vi "nanocal -- nuclear schottky fit V7.vi"() -> ()   [LabVIEW 2021] (continued)
0494_220602_RAW_cal__ref_\" ->   <|    \"ζ\" -> 0.158252879790   ,  \"τ1\" -> 0.024827950008   ,  \"τS\" -> 0.060146890842   ,  \"τN\" -> 0.015050943013   ,  \"τC\" -> 0.000951750255   ,  \"κ0\" -> 0.000000001243   ,  \"mm1\" -> 0.000128517617   ,  \"mm2\" -> 0.018585917114   ,  \"mm3\" -> 0.094163373149   ,  \"T\" -> 0.250000000000   ,  \"B\" -> 8.000000000000   ,  \"θ\" -> 45.000000000000   ,  \"Reoff\" -> -20024489.795918367800   ,  \"Imoff\" -> 0.000000000000   ,  \"στ1\" -> 0.008614865267   ,  \"στS\" -> 0.002364789587   ,  \"στN\" -> 0.002490160339    |>   , \n\"IDS0494_220602_RAW_cal__sam_\" ->   <|    \"ζ\" -> 0.000000000000   ,  \"τ1\" -> 0.000000000000   ,  \"τS\" -> 0.000000000000   ,  \"τN\" -> 0.000000000000   ,  \"τC\" -> 0.000000000000   ,  \"κ0\" -> 0.000000000000   ,  \"mm1\" -> 0.000000000000   ,  \"mm2\" -> 0.000000000000   ,  \"mm3\" -> 0.000000000000   ,  \"T\" -> 0.250000000000   ,  \"B\" -> 8.000000000000   ,  \"θ\" -> 45.000000000000   ,  \"Reoff\" -> 0.000000000000   ,  \"Imoff\" -> 0.000000000000   ,  \"στ1\" -> 0.000000000000   ,  \"στS\" -> 0.000000000000   ,  \"στN\" -> 0.000000000000    |>   , \n\"IDS0495_220602_RAW_cal__ref_\" ->   <|    \"ζ\" -> 0.620326639374   ,  \"τ1\" -> 0.043464597459   ,  \"τS\" -> 0.134106398601   ,  \"τN\" -> 0.331630286291   ,  \"τC\" -> 0.000791545838   ,  \"κ0\" -> 0.000000000449   ,  \"mm1\" -> 0.000302343125   ,  \"mm2\" -> 0.012035033998   ,  \"mm3\" -> 0.786564323638   ,  \"T\" -> 0.120000000000   ,  \"B\" -> 8.000000000000   ,  \"θ\" -> 45.000000000000   ,  \"Reoff\" -> -197355102.040816367000   ,  \"Imoff\" -> 0.000000000000   ,  \"στ1\" -> 0.040479747535   ,  \"στS\" -> 0.067583774677   ,  \"στN\" -> 0.126300079114    |>   , \n\"IDS0495_220602_RAW_cal__sam_\" ->   <|    \"ζ\" -> 0.000000000000   ,  \"τ1\" -> 0.000000000000   ,  \"τS\" -> 0.000000000000   ,  \"τN\" -> 0.000000000000   ,  \"τC\" -> 0.000000000000   ,  \"κ0\" -> 0.000000000000   ,  \"mm1\" -> 0.000000000000   ,  \"mm2\" -> 0.000000000000   ,  \"mm3\" -> 0.000000000000   ,  \"T\" -> 0.120000000000   ,  \"B\" -> 8.000000000000   ,  \"θ\" -> 45.000000000000   ,  \"Reoff\" -> 0.000000000000   ,  \"Imoff\" -> 0.000000000000   ,  \"στ1\" -> 0.000000000000   ,  \"στS\" -> 0.000000000000   ,  \"στN\" -> 0.000000000000    |>   , \n\"IDS0496_220602_RAW_cal__ref_\" ->   <|    \"ζ\" -> 0.427468854343   ,  \"τ1\" -> 0.039705721457   ,  \"τS\" -> 0.111520336177   ,  \"τN\" -> 0.118737423491   ,  \"τC\" -> 0.000757643682   ,  \"κ0\" -> 0.000000000613   ,  \"mm1\" -> 0.000226123834   ,  \"mm2\" -> 0.018076446652   ,  \"mm3\" -> 0.350846575050   ,  \"T\" -> 0.150000000000   ,  \"B\" -> 8.000000000000   ,  \"θ\" -> 45.000000000000   ,  \"Reoff\" -> -103289795.918367386000   ,  \"Imoff\" -> 0.000000000000   ,  \"στ1\" -> 0.024554050195   ,  \"στS\" -> 0.027075430846   ,  \"στN\" -> 0.033199054106    |>   , \n\"IDS0496_220602_RAW_cal__sam_\" ->   <|    \"ζ\" -> 0.000000000000   ,  \"τ1\" -> 0.000000000000   ,  \"τS\" -> 0.000000000000   ,  \"τN\" -> 0.000000000000   ,  \"τC\" -> 0.000000000000   ,  \"κ0\" -> 0.000000000000   ,  \"mm1\" -> 0.000000000000   ,  \"mm2\" -> 0.000000000000   ,  \"mm3\" -> 0.000000000000   ,  \"T\" -> 0.150000000000   ,  \"B\" -> 8.000000000000   ,  \"θ\" -> 45.000000000000   ,  \"Reoff\" -> 0.000000000000   ,  \"Imoff\" -> 0.000000000000   ,  \"στ1\" -> 0.000000000000   ,  \"στS\" -> 0.000000000000   ,  \"στN\" -> 0.000000000000    |>   , \n\"IDS0497_220603_RAW_cal__ref_\" ->   <|    \"ζ\" -> 0.332403347952   ,  \"τ1\" -> 0.033892588666   ,  \"τS\" -> 0.089882476524   ,  \"τN\" -> 0.072116867912   ,  \"τC\" -> 0.000736636997   ,  \"κ0\" -> 0.000000000736   ,  \"mm1\" -> 0.000182924179   ,  \"mm2\" -> 0.017518148856   ,  \"mm3\" -> 0.232776621520   ,  \"T\" -> 0.170000000000   ,  \"B\" -> 8.000000000000   ,  \"θ\" -> 45.000000000000   ,  \"Reoff\" -> -72616326.530612289900   ,  \"Imoff\" -> 0.000000000000   ,  \"στ1\" -> 0.010864544003   ,  \"στS\" -> 0.009543194360   ,  \"στN\" -> 0.010830263954    |>   , \n\"IDS0497_220603_RAW_cal__sam_\" ->   <|    \"ζ\" -> 0.000000000000   ,  \"τ1\" -> 0.000000000000   ,  \"τS\" -> 0.000000000000   ,  \"τN\" -> 0.000000000000   ,  \"τC\" -> 0.000000000000   ,  \"κ0\" -> 0.000000000000   ,  \"mm1\" -> 0.000000000000   ,  \"mm2\" -> 0.000000000000   ,  \"mm3\" -> 0.000000000000   ,  \"T\" -> 0.170000000000   ,  \"B\" -> 8.000000000000   ,  \"θ\" -> 45.000000000000   ,  \"Reoff\" -> 0.000000000000   ,  \"Imoff\" -> 0.000000000000   ,  \"στ1\" -> 0.000000000000   ,  \"στS\" -> 0.000000000000   ,  \"στN\" -> 0.000000000000    |>   , \n\"IDS0498_220603_RAW_cal__ref_\" ->   <|    \"ζ\" -> 0.110734162984   ,  \"τ1\" -> 0.019381596449   ,  \"τS\" -> 0.049800010244   ,  \"τN\" -> 0.007874153241   ,  \"τC\" -> 0.001094666009   ,  \"κ0\" -> 0.000000001580   ,  \"mm1\" -> 0.000107216591   ,  \"mm2\" -> 0.015930752272   ,  \"mm3\" -> 0.068498957299   ,  \"T\" -> 0.300000000000   ,  \"B\" -> 8.000000000000   ,  \"θ\" -> 45.000000000000   ,  \"Reoff\" -> -10657142.857142858200   ,  \"Imoff\" -> 0.000000000000   ,  \"στ1\" -> 0.007394501349   ,  \"στS\" -> 0.001744107422   ,  \"στN\" -> 0.001987690041    |>   , \n\"IDS0498_220603_RAW_cal__sam_\" ->   <|    \"ζ\" -> 0.000000000000   ,  \"τ1\" -> 0.000000000000   ,  \"τS\" -> 0.000000000000   ,  \"τN\" -> 0.000000000000   ,  \"τC\" -> 0.000000000000   ,  \"κ0\" -> 0.000000000000   ,  \"mm1\" -> 0.000000000000   ,  \"mm2\" -> 0.000000000000   ,  \"mm3\" -> 0.000000000000   ,  \"T\" -> 0.300000000000   ,  \"B\" -> 8.000000000000   ,  \"θ\" -> 45.000000000000   ,  \"Reoff\" -> 0.000000000000   ,  \"Imoff\" -> 0.000000000000   ,  \"στ1\" -> 0.000000000000   ,  \"στS\" -> 0.000000000000   ,  \"στN\" -> 0.000000000000    |>   , \n\"IDS0499_220603_RAW_cal__ref_\" ->   <|    \"ζ\" -> 0.075729964973   ,  \"τ1\" -> 0.017492157350   ,  \"τS\" -> 0.042916924435   ,  \"τN\" -> 0.003910009488   ,  \"τC\" -> 0.001485143735   ,  \"κ0\" -> 0.000000001996   ,  \"mm1\" -> 0.000101508308   ,  \"mm2\" -> 0.015465208626   ,  \"mm3\" -> 0.053783720140   ,  \"T\" -> 0.360000000000   ,  \"B\" -> 8.000000000000   ,  \"θ\" -> 45.000000000000   ,  \"Reoff\" -> -3787755.102040812380   ,  \"Imoff\" -> 0.000000000000   ,  \"στ1\" -> 0.001180089795   ,  \"στS\" -> 0.000447730504   ,  \"στN\" -> 0.000150733035    |>   , \n\"IDS0499_220603_RAW_cal__sam_\" ->   <|    \"ζ\" -> 0.000000000000   ,  \"τ1\" -> 0.000000000000   ,  \"τS\" -> 0.000000000000   ,  \"τN\" -> 0.000000000000   ,  \"τC\" -> 0.000000000000   ,  \"κ0\" -> 0.000000000000   ,  \"mm1\" -> 0.000000000000   ,  \"mm2\" -> 0.000000000000   ,  \"mm3\" -> 0.000000000000   ,  \"T\" -> 0.360000000000   ,  \"B\" -> 8.000000000000   ,  \"θ\" -> 45.000000000000   ,  \"Reoff\" -> 0.000000000000   ,  \"Imoff\" -> 0.000000000000   ,  \"στ1\" -> 0.000000000000   ,  \"στS\" -> 0.000000000000   ,  \"στN\" -> 0.000000000000    |>   , \n\"IDS0500_220603_RAW_cal__ref_\" ->   <|    \"ζ\" -> 0.057062025730   ,  \"τ1\" -> 0.015621328716   ,  \"τS\" -> 0.037684759429   ,  \"τN\" -> 0.002528358408   ,  \"τC\" -> 0.001814587656   ,  \"κ0\" -> 0.000000002409   ,  \"mm1\" -> 0.000093897005   ,  \"mm2\" -> 0.014229954054   ,  \"mm3\" -> 0.045619825114   ,  \"T\" -> 0.420000000000   ,  \"B\" -> 8.000000000000   ,  \"θ\" -> 45.000000000000   ,  \"Reoff\" -> -1914285.714285716420   ,  \"Imoff\" -> 0.000000000000   ,  \"στ1\" -> 0.000955516526   ,  \"στS\" -> 0.000234895501   ,  \"στN\" -> 0.000135281330    |>   , \n\"IDS0500_220603_RAW_cal__sam_\" ->   <|    \"ζ\" -> 0.000000000000   ,  \"τ1\" -> 0.000000000000   ,  \"τS\" -> 0.000000000000   ,  \"τN\" -> 0.000000000000   ,  \"τC\" -> 0.000000000000   ,  \"κ0\" -> 0.000000000000   ,  \"mm1\" -> 0.000000000000   ,  \"mm2\" -> 0.000000000000   ,  \"mm3\" -> 0.000000000000   ,  \"T\" -> 0.420000000000   ,  \"B\" -> 8.000000000000   ,  \"θ\" -> 45.000000000000   ,  \"Reoff\" -> 0.000000000000   ,  \"Imoff\" -> 0.000000000000   ,  \"στ1\" -> 0.000000000000   ,  \"στS\" -> 0.000000000000   ,  \"στN\" -> 0.000000000000    |>   , \n\"IDS0501_220603_RAW_cal__ref_\" ->   <|    \"ζ\" -> 0.041820610943   ,  \"τ1\" -> 0.014727705147   ,  \"τS\" -> 0.032103066270   ,  \"τN\" -> 0.001402697929   ,  \"τC\" -> 0.002062288671   ,  \"κ0\" -> 0.000000003070   ,  \"mm1\" -> 0.000078146988   ,  \"mm2\" -> 0.013796091461   ,  \"mm3\" -> 0.037822751096   ,  \"T\" -> 0.520000000000   ,  \"B\" -> 8.000000000000   ,  \"θ\" -> 45.000000000000   ,  \"Reoff\" -> -1155102.040816326160   ,  \"Imoff\" -> 0.000000000000   ,  \"στ1\" -> 0.000294282186   ,  \"στS\" -> 0.000104705305   ,  \"στN\" -> 0.000024302938    |>   , \n\"IDS0501_220603_RAW_cal__sam_\" ->   <|    \"ζ\" -> 0.000000000000   ,  \"τ1\" -> 0.000000000000   ,  \"τS\" -> 0.000000000000   ,  \"τN\" -> 0.000000000000   ,  \"τC\" -> 0.000000000000   ,  \"κ0\" -> 0.000000000000   ,  \"mm1\" -> 0.000000000000   ,  \"mm2\" -> 0.000000000000   ,  \"mm3\" -> 0.000000000000   ,  \"T\" -> 0.520000000000   ,  \"B\" -> 8.000000000000   ,  \"θ\" -> 45.000000000000   ,  \"Reoff\" -> 0.000000000000   ,  \"Imoff\" -> 0.000000000000   ,  \"στ1\" -> 0.000000000000   ,  \"στS\" -> 0.000000000000   ,  \"στN\" -> 0.000000000000    |>   , \n\"IDS0502_220603_RAW_cal__ref_\" ->   <|    \"ζ\" -> 0.034670986979   ,  \"τ1\" -> 0.014178027620   ,  \"τS\" -> 0.028243061757   ,  \"τN\" -> 0.000956770293   ,  \"τC\" -> 0.002118106957   ,  \"κ0\" -> 0.000000003766   ,  \"mm1\" -> 0.000066318852   ,  \"mm2\" -> 0.013432939767   ,  \"mm3\" -> 0.033009095005   ,  \"T\" -> 0.620000000000   ,  \"B\" -> 8.000000000000   ,  \"θ\" -> 45.000000000000   ,  \"Reoff\" -> -1228571.428571428170   ,  \"Imoff\" -> 0.000000000000   ,  \"στ1\" -> 0.000460475840   ,  \"στS\" -> 0.000103102463   ,  \"στN\" -> 0.000021520778    |>   , \n\"IDS0502_220603_RAW_cal__sam_\" ->   <|    \"ζ\" -> 0.000000000000   ,  \"τ1\" -> 0.000000000000   ,  \"τS\" -> 0.000000000000   ,  \"τN\" -> 0.000000000000   ,  \"τC\" -> 0.000000000000   ,  \"κ0\" -> 0.000000000000   ,  \"mm1\" -> 0.000000000000   ,  \"mm2\" -> 0.000000000000   ,  \"mm3\" -> 0.000000000000   ,  \"T\" -> 0.620000000000   ,  \"B\" -> 8.000000000000   ,  \"θ\" -> 45.000000000000   ,  \"Reoff\" -> 0.000000000000   ,  \"Imoff\" -> 0.000000000000   ,  \"στ1\" -> 0.000000000000   ,  \"στS\" -> 0.000000000000   ,  \"στN\" -> 0.000000000000    |>   , \n\"IDS0503_220603_RAW_cal__ref_\" ->   <|    \"ζ\" -> 0.027095379561   ,  \"τ1\" -> 0.013653054815   ,  \"τS\" -> 0.022995805893   ,  \"τN\" -> 0.000444319703   ,  \"τC\" -> 0.002402226581   ,  \"κ0\" -> 0.000000005139   ,  \"mm1\" -> 0.000057649030   ,  \"mm2\" -> 0.013182559678   ,  \"mm3\" -> 0.026890317385   ,  \"T\" -> 0.820000000000   ,  \"B\" -> 8.000000000000   ,  \"θ\" -> 45.000000000000   ,  \"Reoff\" -> -959183.673469387459   ,  \"Imoff\" -> 0.000000000000   ,  \"στ1\" -> 0.001867148954   ,  \"στS\" -> 0.000121343744   ,  \"στN\" -> 0.000029055500    |>   , \n\"IDS0503_220603_RAW_cal__sam_\" ->   <|    \"ζ\" -> 0.000000000000   ,  \"τ1\" -> 0.000000000000   ,  \"τS\" -> 0.000000000000   ,  \"τN\" -> 0.000000000000   ,  \"τC\" -> 0.000000000000   ,  \"κ0\" -> 0.000000000000   ,  \"mm1\" -> 0.000000000000   ,  \"mm2\" -> 0.000000000000   ,  \"mm3\" -> 0.000000000000   ,  \"T\" -> 0.820000000000   ,  \"B\" -> 8.000000000000   ,  \"θ\" -> 45.000000000000   ,  \"Reoff\" -> 0.000000000000   ,  \"Imoff\" -> 0.000000000000   ,  \"στ1\" -> 0.000000000000   ,  \"στS\" -> 0.000000000000   ,  \"στN\" -> 0.000000000000    |>   , \n\"IDS0504_220603_RAW_cal__ref_\" ->   <|    \"ζ\" -> 0.022447798358   ,  \"τ1\" -> 0.013732237823   ,  \"τS\" -> 0.018577417913   ,  \"τN\" -> 0.000173926586   ,  \"τC\" -> 0.002459582749   ,  \"κ0\" -> 0.000000007201   ,  \"mm1\" -> 0.000047916077   ,  \"mm2\" -> 0.013432779765   ,  \"mm3\" -> 0.021883395630   ,  \"T\" -> 1.120000000000   ,  \"B\" -> 8.000000000000   ,  \"θ\" -> 45.000000000000   ,  \"Reoff\" -> -714285.714285713619   ,  \"Imoff\" -> 0.000000000000   ,  \"στ1\" -> 0.000607993232   ,  \"στS\" -> 0.000105526265   ,  \"στN\" -> 0.000003332790    |>   , \n\"IDS0504_220603_RAW_cal__sam_\" ->   <|    \"ζ\" -> 0.000000000000   ,  \"τ1\" -> 0.000000000000   ,  \"τS\" -> 0.000000000000   ,  \"τN\" -> 0.000000000000   ,  \"τC\" -> 0.000000000000   ,  \"κ0\" -> 0.000000000000   ,  \"mm1\" -> 0.000000000000   ,  \"mm2\" -> 0.000000000000   ,  \"mm3\" -> 0.000000000000   ,  \"T\" -> 1.120000000000   ,  \"B\" -> 8.000000000000   ,  \"θ\" -> 45.000000000000   ,  \"Reoff\" -> 0.000000000000   ,  \"Imoff\" -> 0.000000000000   ,  \"στ1\" -> 0.000000000000   ,  \"στS\" -> 0.000000000000   ,  \"στN\" -> 0.000000000000    |>   , \n\"IDS0505_220603_RAW_cal__ref_\" ->   <|    \"ζ\" -> 0.017603951649   ,  \"τ1\" -> 0.013742471601   ,  \"τS\" -> 0.012869162108   ,  \"τN\" -> 0.000062251305   ,  \"τC\" -> 0.002783258647   ,  \"κ0\" -> 0.000000012669   ,  \"mm1\" -> 0.000039808958   ,  \"mm2\" -> 0.013395445115   ,  \"mm3\" -> 0.016249533565   ,  \"T\" -> 1.900000000000   ,  \"B\" -> 8.000000000000   ,  \"θ\" -> 45.000000000000   ,  \"Reoff\" -> -322448.979591836221   ,  \"Imoff\" -> 0.000000000000   ,  \"στ1\" -> 0.000975208988   ,  \"στS\" -> 0.000083582947   ,  \"στN\" -> 0.000002846022    |>   , \n\"IDS0505_220603_RAW_cal__sam_\" ->   <|    \"ζ\" -> 0.000000000000   ,  \"τ1\" -> 0.000000000000   ,  \"τS\" -> 0.000000000000   ,  \"τN\" -> 0.000000000000   ,  \"τC\" -> 0.000000000000   ,  \"κ0\" -> 0.000000000000   ,  \"mm1\" -> 0.000000000000   ,  \"mm2\" -> 0.000000000000   ,  \"mm3\" -> 0.000000000000   ,  \"T\" -> 1.900000000000   ,  \"B\" -> 8.000000000000   ,  \"θ\" -> 45.000000000000   ,  \"Reoff\" -> 0.000000000000   ,  \"Imoff\" -> 0.000000000000   ,  \"στ1\" -> 0.000000000000   ,  \"στS\" -> 0.000000000000   ,  \"στN\" -> 0.000000000000    |>   , \n\"IDS0506_220603_RAW_cal__ref_\" ->   <|    \"ζ\" -> 0.017513535650   ,  \"τ1\" -> 0.013742433942   ,  \"τS\" -> 0.009294247030   ,  \"τN\" -> 0.000023643269   ,  \"τC\" -> 0.002563999230   ,  \"κ0\" -> 0.000000022469   ,  \"mm1\" -> 0.000034819598   ,  \"mm2\" -> 0.011836880672   ,  \"mm3\" -> 0.013915812404   ,  \"T\" -> 3.100000000000   ,  \"B\" -> 8.000000000000   ,  \"θ\" -> 45.000000000000   ,  \"Reoff\" -> -175510.204081632197   ,  \"Imoff\" -> 0.000000000000   ,  \"στ1\" -> 0.000768522779   ,  \"στS\" -> 0.000063413326   ,  \"στN\" -> 0.000000634158    |>   , \n\"IDS0506_220603_RAW_cal__sam_\" ->   <|    \"ζ\" -> 0.000000000000   ,  \"τ1\" -> 0.000000000000   ,  \"τS\" -> 0.000000000000   ,  \"τN\" -> 0.000000000000   ,  \"τC\" -> 0.000000000000   ,  \"κ0\" -> 0.000000000000   ,  \"mm1\" -> 0.000000000000   ,  \"mm2\" -> 0.000000000000   ,  \"mm3\" -> 0.000000000000   ,  \"T\" -> 3.100000000000   ,  \"B\" -> 8.000000000000   ,  \"θ\" -> 45.000000000000   ,  \"Reoff\" -> 0.000000000000   ,  \"Imoff\" -> 0.000000000000   ,  \"στ1\" -> 0.000000000000   ,  \"στS\" -> 0.000000000000   ,  \"στN\" -> 0.000000000000    |>   , \n\"IDS0508_220603_RAW_cal__ref_\" ->   <|    \"ζ\" -> 0.243281471751   ,  \"τ1\" -> 0.025048654847   ,  \"τS\" -> 0.062611130643   ,  \"τN\" -> 0.020042988527   ,  \"τC\" -> 0.000849297815   ,  \"κ0\" -> 0.000000000907   ,  \"mm1\" -> 0.000164736185   ,  \"mm2\" -> 0.017764187201   ,  \"mm3\" -> 0.110731364203   ,  \"T\" -> 0.200000000000   ,  \"B\" -> 6.000000000000   ,  \"θ\" -> 45.000000000000   ,  \"Reoff\" -> -40636734.693877548000   ,  \"Imoff\" -> 0.000000000000   ,  \"στ1\" -> 0.014234353727   ,  \"στS\" -> 0.004838976210   ,  \"στN\" -> 0.004976250052    |>   , \n\"IDS0508_220603_RAW_cal__sam_\" ->   <|    \"ζ\" -> 0.000000000000   ,  \"τ1\" -> 0.000000000000   ,  \"τS\" -> 0.000000000000   ,  \"τN\" -> 0.000000000000   ,  \"τC\" -> 0.000000000000   ,  \"κ0\" -> 0.000000000000   ,  \"mm1\" -> 0.000000000000   ,  \"mm2\" -> 0.000000000000   ,  \"mm3\" -> 0.000000000000   ,  \"T\" -> 0.200000000000   ,  \"B\" -> 6.000000000000   ,  \"θ\" -> 45.000000000000   ,  \"Reoff\" -> 0.000000000000   ,  \"Imoff\" -> 0.000000000000   ,  \"στ1\" -> 0.000000000000   ,  \"στS\" -> 0.000000000000   ,  \"στN\" -> 0.000000000000    |>   , \n\"IDS0509_220603_RAW_cal__ref_\" ->   <|    \"ζ\" -> 0.413507557358   ,  \"τ1\" -> 0.033675995603   ,  \"τS\" -> 0.093816108912   ,  \"τN\" -> 0.061390510422   ,  \"τC\" -> 0.000803159189   ,  \"κ0\" -> 0.000000000612   ,  \"mm1\" -> 0.000233947412   ,  \"mm2\" -> 0.019125451380   ,  \"mm3\" -> 0.234505485381   ,  \"T\" -> 0.150000000000   ,  \"B\" -> 6.000000000000   ,  \"θ\" -> 45.000000000000   ,  \"Reoff\" -> -88975510.204081654600   ,  \"Imoff\" -> 0.000000000000   ,  \"στ1\" -> 0.030359635336   ,  \"στS\" -> 0.022777334435   ,  \"στN\" -> 0.025753606266    |>   , \n\"IDS0509_220603_RAW_cal__sam_\" ->   <|    \"ζ\" -> 0.000000000000   ,  \"τ1\" -> 0.000000000000   ,  \"τS\" -> 0.000000000000   ,  \"τN\" -> 0.000000000000   ,  \"τC\" -> 0.000000000000   ,  \"κ0\" -> 0.000000000000   ,  \"mm1\" -> 0.000000000000   ,  \"mm2\" -> 0.000000000000   ,  \"mm3\" -> 0.000000000000   ,  \"T\" -> 0.150000000000   ,  \"B\" -> 6.000000000000   ,  \"θ\" -> 45.000000000000   ,  \"Reoff\" -> 0.000000000000   ,  \"Imoff\" -> 0.000000000000   ,  \"στ1\" -> 0.000000000000   ,  \"στS\" -> 0.000000000000   ,  \"στN\" -> 0.000000000000    |>   , \n\"IDS0510_220603_RAW_cal__ref_\" ->   <|    \"ζ\" -> 0.613284276562   ,  \"τ1\" -> 0.039588841090   ,  \"τS\" -> 0.126363579952   ,  \"τN\" -> 0.150529821612   ,  \"τC\" -> 0.000834158039   ,  \"κ0\" -> 0.000000000449   ,  \"mm1\" -> 0.000316290952   ,  \"mm2\" -> 0.017230786632   ,  \"mm3\" -> 0.469583692571   ,  \"T\" -> 0.120000000000   ,  \"B\" -> 6.000000000000   ,  \"θ\" -> 45.000000000000   ,  \"Reoff\" -> -183040816.326530635000   ,  \"Imoff\" -> 0.000000000000   ,  \"στ1\" -> 0.058972518993   ,  \"στS\" -> 0.069910296081   ,  \"στN\" -> 0.097464298744    |>   , \n\"IDS0510_220603_RAW_cal__sam_\" ->   <|    \"ζ\" -> 0.000000000000   ,  \"τ1\" -> 0.000000000000   ,  \"τS\" -> 0.000000000000   ,  \"τN\" -> 0.000000000000   ,  \"τC\" -> 0.000000000000   ,  \"κ0\" -> 0.000000000000   ,  \"mm1\" -> 0.000000000000   ,  \"mm2\" -> 0.000000000000   ,  \"mm3\" -> 0.000000000000   ,  \"T\" -> 0.120000000000   ,  \"B\" -> 6.000000000000   ,  \"θ\" -> 45.000000000000   ,  \"Reoff\" -> 0.000000000000   ,  \"Imoff\" -> 0.000000000000   ,  \"στ1\" -> 0.000000000000   ,  \"στS\" -> 0.000000000000   ,  \"στN\" -> 0.000000000000    |>   , \n\"IDS0511_220604_RAW_cal__ref_\" ->   <|    \"ζ\" -> 0.330310083388   ,  \"τ1\" -> 0.030298910704   ,  \"τS\" -> 0.075236256272   ,  \"τN\" -> 0.040258490760   ,  \"τC\" -> 0.000782924983   ,  \"κ0\" -> 0.000000000728   ,  \"mm1\" -> 0.000193254303   ,  \"mm2\" -> 0.018356930637   ,  \"mm3\" -> 0.166175477301   ,  \"T\" -> 0.170000000000   ,  \"B\" -> 6.000000000000   ,  \"θ\" -> 45.000000000000   ,  \"Reoff\" -> -64436734.693877577800   ,  \"Imoff\" -> 0.000000000000   ,  \"στ1\" -> 0.014626951982   ,  \"στS\" -> 0.008056203133   ,  \"στN\" -> 0.008938953770    |>   , \n\"IDS0511_220604_RAW_cal__sam_\" ->   <|    \"ζ\" -> 0.000000000000   ,  \"τ1\" -> 0.000000000000   ,  \"τS\" -> 0.000000000000   ,  \"τN\" -> 0.000000000000   ,  \"τC\" -> 0.000000000000   ,  \"κ0\" -> 0.000000000000   ,  \"mm1\" -> 0.000000000000   ,  \"mm2\" -> 0.000000000000   ,  \"mm3\" -> 0.000000000000   ,  \"T\" -> 0.170000000000   ,  \"B\" -> 6.000000000000   ,  \"θ\" -> 45.000000000000   ,  \"Reoff\" -> 0.000000000000   ,  \"Imoff\" -> 0.000000000000   ,  \"στ1\" -> 0.000000000000   ,  \"στS\" -> 0.000000000000   ,  \"στN\" -> 0.000000000000    |>   , \n\"IDS0512_220604_RAW_cal__ref_\" ->   <|    \"ζ\" -> 0.157633362112   ,  \"τ1\" -> 0.020861334985   ,  \"τS\" -> 0.051508696686   ,  \"τN\" -> 0.008332770174   ,  \"τC\" -> 0.001009053466   ,  \"κ0\" -> 0.000000001248   ,  \"mm1\" -> 0.000135415312   ,  \"mm2\" -> 0.017070380875   ,  \"mm3\" -> 0.073939070739   ,  \"T\" -> 0.250000000000   ,  \"B\" -> 6.000000000000   ,  \"θ\" -> 45.000000000000   ,  \"Reoff\" -> -16726530.612244904000   ,  \"Imoff\" -> 0.000000000000   ,  \"στ1\" -> 0.019204175583   ,  \"στS\" -> 0.003261272874   ,  \"στN\" -> 0.003231373649    |>   , \n\"IDS0512_220604_RAW_cal__sam_\" ->   <|    \"ζ\" -> 0.000000000000   ,  \"τ1\" -> 0.000000000000   ,  \"τS\" -> 0.000000000000   ,  \"τN\" -> 0.000000000000   ,  \"τC\" -> 0.000000000000   ,  \"κ0\" -> 0.000000000000   ,  \"mm1\" -> 0.000000000000   ,  \"mm2\" -> 0.000000000000   ,  \"mm3\" -> 0.000000000000   ,  \"T\" -> 0.250000000000   ,  \"B\" -> 6.000000000000   ,  \"θ\" -> 45.000000000000   ,  \"Reoff\" -> 0.000000000000   ,  \"Imoff\" -> 0.000000000000   ,  \"στ1\" -> 0.000000000000   ,  \"στS\" -> 0.000000000000   ,  \"στN\" -> 0.000000000000    |>   , \n\"IDS0513_220604_RAW_cal__ref_\" ->   <|    \"ζ\" -> 0.109354643265   ,  \"τ1\" -> 0.019745794663   ,  \"τS\" -> 0.045929868636   ,  \"τN\" -> 0.004362632792   ,  \"τC\" -> 0.001089331798   ,  \"κ0\" -> 0.000000001568   ,  \"mm1\" -> 0.000105345441   ,  \"mm2\" -> 0.017323789537   ,  \"mm3\" -> 0.059198211464   ,  \"T\" -> 0.300000000000   ,  \"B\" -> 6.000000000000   ,  \"θ\" -> 45.000000000000   ,  \"Reoff\" -> -9718367.346938773990   ,  \"Imoff\" -> 0.000000000000   ,  \"στ1\" -> 0.000746121350   ,  \"στS\" -> 0.000145078797   ,  \"στN\" -> 0.000139513521    |>   , \n\"IDS0513_220604_RAW_cal__sam_\" ->   <|    \"ζ\" -> 0.000000000000   ,  \"τ1\" -> 0.000000000000   ,  \"τS\" -> 0.000000000000   ,  \"τN\" -> 0.000000000000   ,  \"τC\" -> 0.000000000000   ,  \"κ0\" -> 0.000000000000   ,  \"mm1\" -> 0.000000000000   ,  \"mm2\" -> 0.000000000000   ,  \"mm3\" -> 0.000000000000   ,  \"T\" -> 0.300000000000   ,  \"B\" -> 6.000000000000   ,  \"θ\" -> 45.000000000000   ,  \"Reoff\" -> 0.000000000000   ,  \"Imoff\" -> 0.000000000000   ,  \"στ1\" -> 0.000000000000   ,  \"στS\" -> 0.000000000000   ,  \"στN\" -> 0.000000000000    |>   , \n\"IDS0514_220604_RAW_cal__ref_\" ->   <|    \"ζ\" -> 0.078464971050   ,  \"τ1\" -> 0.017563831776   ,  \"τS\" -> 0.042315631100   ,  \"τN\" -> 0.002449698464   ,  \"τC\" -> 0.001311085354   ,  \"κ0\" -> 0.000000001978   ,  \"mm1\" -> 0.000092908726   ,  \"mm2\" -> 0.016171593309   ,  \"mm3\" -> 0.050888254947   ,  \"T\" -> 0.360000000000   ,  \"B\" -> 6.000000000000   ,  \"θ\" -> 45.000000000000   ,  \"Reoff\" -> -5555102.040816326630   ,  \"Imoff\" -> 0.000000000000   ,  \"στ1\" -> 0.001705710692   ,  \"στS\" -> 0.000224693737   ,  \"στN\" -> 0.000168766252    |>   , \n\"IDS0514_220604_RAW_cal__sam_\" ->   <|    \"ζ\" -> 0.000000000000   ,  \"τ1\" -> 0.000000000000   ,  \"τS\" -> 0.000000000000   ,  \"τN\" -> 0.000000000000   ,  \"τC\" -> 0.000000000000   ,  \"κ0\" -> 0.000000000000   ,  \"mm1\" -> 0.000000000000   ,  \"mm2\" -> 0.000000000000   ,  \"mm3\" -> 0.000000000000   ,  \"T\" -> 0.360000000000   ,  \"B\" -> 6.000000000000   ,  \"θ\" -> 45.000000000000   ,  \"Reoff\" -> 0.000000000000   ,  \"Imoff\" -> 0.000000000000   ,  \"στ1\" -> 0.000000000000   ,  \"στS\" -> 0.000000000000   ,  \"στN\" -> 0.000000000000    |>   , \n\"IDS0515_220604_RAW_cal__ref_\" ->   <|    \"ζ\" -> 0.061585995431   ,  \"τ1\" -> 0.017021907134   ,  \"τS\" -> 0.041190711561   ,  \"τN\" -> 0.001390110365   ,  \"τC\" -> 0.001428995669   ,  \"κ0\" -> 0.000000002390   ,  \"mm1\" -> 0.000080420017   ,  \"mm2\" -> 0.016194561258   ,  \"mm3\" -> 0.047379125758   ,  \"T\" -> 0.430000000000   ,  \"B\" -> 6.000000000000   ,  \"θ\" -> 45.000000000000   ,  \"Reoff\" -> -4253061.224489795980   ,  \"Imoff\" -> 0.000000000000   ,  \"στ1\" -> 0.004152949973   ,  \"στS\" -> 0.000363204682   ,  \"στN\" -> 0.000192260687    |>   , \n\"IDS0515_220604_RAW_cal__sam_\" ->   <|    \"ζ\" -> 0.000000000000   ,  \"τ1\" -> 0.000000000000   ,  \"τS\" -> 0.000000000000   ,  \"τN\" -> 0.000000000000   ,  \"τC\" -> 0.000000000000   ,  \"κ0\" -> 0.000000000000   ,  \"mm1\" -> 0.000000000000   ,  \"mm2\" -> 0.000000000000   ,  \"mm3\" -> 0.000000000000   ,  \"T\" -> 0.430000000000   ,  \"B\" -> 6.000000000000   ,  \"θ\" -> 45.000000000000   ,  \"Reoff\" -> 0.000000000000   ,  \"Imoff\" -> 0.000000000000   ,  \"στ1\" -> 0.000000000000   ,  \"στS\" -> 0.000000000000   ,  \"στN\" -> 0.000000000000    |>   , \n\"IDS0516_220604_RAW_cal__ref_\" ->   <|    \"ζ\" -> 0.045061124228   ,  \"τ1\" -> 0.016174333666   ,  \"τS\" -> 0.041331628225   ,  \"τN\" -> 0.001008746985   ,  \"τC\" -> 0.001666143406   ,  \"κ0\" -> 0.000000003072   ,  \"mm1\" -> 0.000069279556   ,  \"mm2\" -> 0.015610467629   ,  \"mm3\" -> 0.046409010004   ,  \"T\" -> 0.520000000000   ,  \"B\" -> 6.000000000000   ,  \"θ\" -> 45.000000000000   ,  \"Reoff\" -> -2636734.693877550770   ,  \"Imoff\" -> 0.000000000000   ,  \"στ1\" -> 0.000679845630   ,  \"στS\" -> 0.000215440983   ,  \"στN\" -> 0.000036761910    |>   , \n\"IDS0516_220604_RAW_cal__sam_\" ->   <|    \"ζ\" -> 0.000000000000   ,  \"τ1\" -> 0.000000000000   ,  \"τS\" -> 0.000000000000   ,  \"τN\" -> 0.000000000000   ,  \"τC\" -> 0.000000000000   ,  \"κ0\" -> 0.000000000000   ,  \"mm1\" -> 0.000000000000   ,  \"mm2\" -> 0.000000000000   ,  \"mm3\" -> 0.000000000000   ,  \"T\" -> 0.520000000000   ,  \"B\" -> 6.000000000000   ,  \"θ\" -> 45.000000000000   ,  \"Reoff\" -> 0.000000000000   ,  \"Imoff\" -> 0.000000000000   ,  \"στ1\" -> 0.000000000000   ,  \"στS\" -> 0.000000000000   ,  \"στN\" -> 0.000000000000    |>   , \n\"IDS0517_220604_RAW_cal__ref_\" ->   <|    \"ζ\" -> 0.037661249073   ,  \"τ1\" -> 0.016158267438   ,  \"τS\" -> 0.041535470501   ,  \"τN\" -> 0.000589951470   ,  \"τC\" -> 0.001574909889   ,  \"κ0\" -> 0.000000003727   ,  \"mm1\" -> 0.000055213424   ,  \"mm2\" -> 0.015821969361   ,  \"mm3\" -> 0.045567912522   ,  \"T\" -> 0.620000000000   ,  \"B\" -> 6.000000000000   ,  \"θ\" -> 45.000000000000   ,  \"Reoff\" -> -2277551.020408163780   ,  \"Imoff\" -> 0.000000000000   ,  \"στ1\" -> 0.000926762360   ,  \"στS\" -> 0.000192613038   ,  \"στN\" -> 0.000026616394    |>   , \n\"IDS0517_220604_RAW_cal__sam_\" ->   <|    \"ζ\" -> 0.000000000000   ,  \"τ1\" -> 0.000000000000   ,  \"τS\" -> 0.000000000000   ,  \"τN\" -> 0.000000000000   ,  \"τC\" -> 0.000000000000   ,  \"κ0\" -> 0.000000000000   ,  \"mm1\" -> 0.000000000000   ,  \"mm2\" -> 0.000000000000   ,  \"mm3\" -> 0.000000000000   ,  \"T\" -> 0.620000000000   ,  \"B\" -> 6.000000000000   ,  \"θ\" -> 45.000000000000   ,  \"Reoff\" -> 0.000000000000   ,  \"Imoff\" -> 0.000000000000   ,  \"στ1\" -> 0.000000000000   ,  \"στS\" -> 0.000000000000   ,  \"στN\" -> 0.000000000000    |>   , \n\"IDS0518_220604_RAW_cal__ref_\" ->   <|    \"ζ\" -> 0.026897195586   ,  \"τ1\" -> 0.017029322947   ,  \"τS\" -> 0.030300618121   ,  \"τN\" -> 0.000253092893   ,  \"τC\" -> 0.002128020527   ,  \"κ0\" -> 0.000000005137   ,  \"mm1\" -> 0.000052252635   ,  \"mm2\" -> 0.016764147571   ,  \"mm3\" -> 0.033716463424   ,  \"T\" -> 0.820000000000   ,  \"B\" -> 6.000000000000   ,  \"θ\" -> 45.000000000000   ,  \"Reoff\" -> -1020408.163265306500   ,  \"Imoff\" -> 0.000000000000   ,  \"στ1\" -> 0.001120431630   ,  \"στS\" -> 0.000175631796   ,  \"στN\" -> 0.000008557959    |>   , \n\"IDS0518_220604_RAW_cal__sam_\" ->   <|    \"ζ\" -> 0.000000000000   ,  \"τ1\" -> 0.000000000000   ,  \"τS\" -> 0.000000000000   ,  \"τN\" -> 0.000000000000   ,  \"τC\" -> 0.000000000000   ,  \"κ0\" -> 0.000000000000   ,  \"mm1\" -> 0.000000000000   ,  \"mm2\" -> 0.000000000000   ,  \"mm3\" -> 0.000000000000   ,  \"T\" -> 0.820000000000   ,  \"B\" -> 6.000000000000   ,  \"θ\" -> 45.000000000000   ,  \"Reoff\" -> 0.000000000000   ,  \"Imoff\" -> 0.000000000000   ,  \"στ1\" -> 0.000000000000   ,  \"στS\" -> 0.000000000000   ,  \"στN\" -> 0.000000000000    |>   , \n\"IDS0519_220604_RAW_cal__ref_\" ->   <|    \"ζ\" -> 0.022664825895   ,  \"τ1\" -> 0.014721420139   ,  \"τS\" -> 0.018200510248   ,  \"τN\" -> 0.000100851172   ,  \"τC\" -> 0.002380537737   ,  \"κ0\" -> 0.000000007190   ,  \"mm1\" -> 0.000046880798   ,  \"mm2\" -> 0.014490052902   ,  \"mm3\" -> 0.021281182766   ,  \"T\" -> 1.120000000000   ,  \"B\" -> 6.000000000000   ,  \"θ\" -> 45.000000000000   ,  \"Reoff\" -> -795918.367346938698   ,  \"Imoff\" -> 0.000000000000   ,  \"στ1\" -> 0.002006498411   ,  \"στS\" -> 0.000156945460   ,  \"στN\" -> 0.000006591622    |>   , \n\"IDS0519_220604_RAW_cal__sam_\" ->   <|    \"ζ\" -> 0.000000000000   ,  \"τ1\" -> 0.000000000000   ,  \"τS\" -> 0.000000000000   ,  \"τN\" -> 0.000000000000   ,  \"τC\" -> 0.000000000000   ,  \"κ0\" -> 0.000000000000   ,  \"mm1\" -> 0.000000000000   ,  \"mm2\" -> 0.000000000000   ,  \"mm3\" -> 0.000000000000   ,  \"T\" -> 1.120000000000   ,  \"B\" -> 6.000000000000   ,  \"θ\" -> 45.000000000000   ,  \"Reoff\" -> 0.000000000000   ,  \"Imoff\" -> 0.000000000000   ,  \"στ1\" -> 0.000000000000   ,  \"στS\" -> 0.000000000000   ,  \"στN\" -> 0.000000000000    |>   , \n\"IDS0520_220604_RAW_cal__ref_\" ->   <|    \"ζ\" -> 0.017334133227   ,  \"τ1\" -> 0.014742496640   ,  \"τS\" -> 0.012814930706   ,  \"τN\" -> 0.000029321869   ,  \"τC\" -> 0.002644067199   ,  \"κ0\" -> 0.000000012608   ,  \"mm1\" -> 0.000037545170   ,  \"mm2\" -> 0.014397895803   ,  \"mm3\" -> 0.016018019426   ,  \"T\" -> 1.900000000000   ,  \"B\" -> 6.000000000000   ,  \"θ\" -> 45.000000000000   ,  \"Reoff\" -> -346938.775510204955   ,  \"Imoff\" -> 0.000000000000   ,  \"στ1\" -> 0.000944080066   ,  \"στS\" -> 0.000100682155   ,  \"στN\" -> 0.000000473993    |>   , \n\"IDS0520_220604_RAW_cal__sam_\" ->   <|    \"ζ\" -> 0.000000000000   ,  \"τ1\" -> 0.000000000000   ,  \"τS\" -> 0.000000000000   ,  \"τN\" -> 0.000000000000   ,  \"τC\" -> 0.000000000000   ,  \"κ0\" -> 0.000000000000   ,  \"mm1\" -> 0.000000000000   ,  \"mm2\" -> 0.000000000000   ,  \"mm3\" -> 0.000000000000   ,  \"T\" -> 1.900000000000   ,  \"B\" -> 6.000000000000   ,  \"θ\" -> 45.000000000000   ,  \"Reoff\" -> 0.000000000000   ,  \"Imoff\" -> 0.000000000000   ,  \"στ1\" -> 0.000000000000   ,  \"στS\" -> 0.000000000000   ,  \"στN\" -> 0.000000000000    |>   , \n\"IDS0521_220604_RAW_cal__ref_\" ->   <|    \"ζ\" -> 0.016488778700   ,  \"τ1\" -> 0.014739187925   ,  \"τS\" -> 0.009276506923   ,  \"τN\" -> 0.000009013062   ,  \"τC\" -> 0.002584186338   ,  \"κ0\" -> 0.000000022490   ,  \"mm1\" -> 0.000032992550   ,  \"mm2\" -> 0.011941581665   ,  \"mm3\" -> 0.014787426917   ,  \"T\" -> 3.100000000000   ,  \"B\" -> 6.000000000000   ,  \"θ\" -> 45.000000000000   ,  \"Reoff\" -> -167346.938775509596   ,  \"Imoff\" -> 0.000000000000   ,  \"στ1\" -> 0.000306328571   ,  \"στS\" -> 0.000088607277   ,  \"στN\" -> 0.000000155207    |>   , \n\"IDS0521_220604_RAW_cal__sam_\" ->   <|    \"ζ\" -> 0.000000000000   ,  \"τ1\" -> 0.000000000000   ,  \"τS\" -> 0.000000000000   ,  \"τN\" -> 0.000000000000   ,  \"τC\" -> 0.000000000000   ,  \"κ0\" -> 0.000000000000   ,  \"mm1\" -> 0.000000000000   ,  \"mm2\" -> 0.000000000000   ,  \"mm3\" -> 0.000000000000   ,  \"T\" -> 3.100000000000   ,  \"B\" -> 6.000000000000   ,  \"θ\" -> 45.000000000000   ,  \"Reoff\" -> 0.000000000000   ,  \"Imoff\" -> 0.000000000000   ,  \"στ1\" -> 0.000000000000   ,  \"στS\" -> 0.000000000000   ,  \"στN\" -> 0.000000000000    |>   , \n\"IDS0523_220604_RAW_cal__ref_\" ->   <|    \"ζ\" -> 0.248494287035   ,  \"τ1\" -> 0.140471463831   ,  \"τS\" -> 0.029170563772   ,  \"τN\" -> 0.016077523258   ,  \"τC\" -> 0.000858124054   ,  \"κ0\" -> 0.000000000897   ,  \"mm1\" -> 0.000167616779   ,  \"mm2\" -> 0.031344824749   ,  \"mm3\" -> 0.166309124513   ,  \"T\" -> 0.200000000000   ,  \"B\" -> 4.000000000000   ,  \"θ\" -> 45.000000000000   ,  \"Reoff\" -> -41942857.142857194000   ,  \"Imoff\" -> 0.000000000000   ,  \"στ1\" -> 0.163113161678   ,  \"στS\" -> 0.000492211177   ,  \"στN\" -> 0.015881366148    |>   , \n\"IDS0523_220604_RAW_cal__sam_\" ->   <|    \"ζ\" -> 0.000000000000   ,  \"τ1\" -> 0.000000000000   ,  \"τS\" -> 0.000000000000   ,  \"τN\" -> 0.000000000000   ,  \"τC\" -> 0.000000000000   ,  \"κ0\" -> 0.000000000000   ,  \"mm1\" -> 0.000000000000   ,  \"mm2\" -> 0.000000000000   ,  \"mm3\" -> 0.000000000000   ,  \"T\" -> 0.200000000000   ,  \"B\" -> 4.000000000000   ,  \"θ\" -> 45.000000000000   ,  \"Reoff\" -> 0.000000000000   ,  \"Imoff\" -> 0.000000000000   ,  \"στ1\" -> 0.000000000000   ,  \"στS\" -> 0.000000000000   ,  \"στN\" -> 0.000000000000    |>   , \n\"IDS0524_220605_RAW_cal__ref_\" ->   <|    \"ζ\" -> 0.342264426031   ,  \"τ1\" -> 0.148951865550   ,  \"τS\" -> 0.034223286872   ,  \"τN\" -> 0.023114154081   ,  \"τC\" -> 0.000835537193   ,  \"κ0\" -> 0.000000000715   ,  \"mm1\" -> 0.000210189792   ,  \"mm2\" -> 0.036494538053   ,  \"mm3\" -> 0.190044682168   ,  \"T\" -> 0.170000000000   ,  \"B\" -> 4.000000000000   ,  \"θ\" -> 45.000000000000   ,  \"Reoff\" -> -68526530.612244904100   ,  \"Imoff\" -> 0.000000000000   ,  \"στ1\" -> 0.142355896146   ,  \"στS\" -> 0.002021018584   ,  \"στN\" -> 0.017181504971    |>   , \n\"IDS0524_220605_RAW_cal__sam_\" ->   <|    \"ζ\" -> 0.000000000000   ,  \"τ1\" -> 0.000000000000   ,  \"τS\" -> 0.000000000000   ,  \"τN\" -> 0.000000000000   ,  \"τC\" -> 0.000000000000   ,  \"κ0\" -> 0.000000000000   ,  \"mm1\" -> 0.000000000000   ,  \"mm2\" -> 0.000000000000   ,  \"mm3\" -> 0.000000000000   ,  \"T\" -> 0.170000000000   ,  \"B\" -> 4.000000000000   ,  \"θ\" -> 45.000000000000   ,  \"Reoff\" -> 0.000000000000   ,  \"Imoff\" -> 0.000000000000   ,  \"στ1\" -> 0.000000000000   ,  \"στS\" -> 0.000000000000   ,  \"στN\" -> 0.000000000000    |>   , \n\"IDS0525_220605_RAW_cal__ref_\" ->   <|    \"ζ\" -> 0.438280595131   ,  \"τ1\" -> 0.137342772879   ,  \"τS\" -> 0.040264580872   ,  \"τN\" -> 0.033372414925   ,  \"τC\" -> 0.000857425660   ,  \"κ0\" -> 0.000000000589   ,  \"mm1\" -> 0.000258601158   ,  \"mm2\" -> 0.039283249404   ,  \"mm3\" -> 0.204569010116   ,  \"T\" -> 0.150000000000   ,  \"B\" -> 4.000000000000   ,  \"θ\" -> 45.000000000000   ,  \"Reoff\" -> -86930612.244897961600   ,  \"Imoff\" -> 0.000000000000   ,  \"στ1\" -> 0.199442289109   ,  \"στS\" -> 0.005269413629   ,  \"στN\" -> 0.036619051524    |>   , \n\"IDS0525_220605_RAW_cal__sam_\" ->   <|    \"ζ\" -> 0.000000000000   ,  \"τ1\" -> 0.000000000000   ,  \"τS\" -> 0.000000000000   ,  \"τN\" -> 0.000000000000   ,  \"τC\" -> 0.000000000000   ,  \"κ0\" -> 0.000000000000   ,  \"mm1\" -> 0.000000000000   ,  \"mm2\" -> 0.000000000000   ,  \"mm3\" -> 0.000000000000   ,  \"T\" -> 0.150000000000   ,  \"B\" -> 4.000000000000   ,  \"θ\" -> 45.000000000000   ,  \"Reoff\" -> 0.000000000000   ,  \"Imoff\" -> 0.000000000000   ,  \"στ1\" -> 0.000000000000   ,  \"στS\" -> 0.000000000000   ,  \"στN\" -> 0.000000000000    |>   , \n\"IDS0526_220605_RAW_cal__ref_\" ->   <|    \"ζ\" -> 0.681535842582   ,  \"τ1\" -> 0.096440830636   ,  \"τS\" -> 0.049346041453   ,  \"τN\" -> 0.056139024949   ,  \"τC\" -> 0.000822867948   ,  \"κ0\" -> 0.000000000444   ,  \"mm1\" -> 0.000331542094   ,  \"mm2\" -> 0.033417308945   ,  \"mm3\" -> 0.240891767557   ,  \"T\" -> 0.120000000000   ,  \"B\" -> 4.000000000000   ,  \"θ\" -> 45.000000000000   ,  \"Reoff\" -> -183040816.326530635000   ,  \"Imoff\" -> 0.000000000000   ,  \"στ1\" -> 0.106020317496   ,  \"στS\" -> 0.010756317478   ,  \"στN\" -> 0.041433473525    |>   , \n\"IDS0526_220605_RAW_cal__sam_\" ->   <|    \"ζ\" -> 0.000000000000   ,  \"τ1\" -> 0.000000000000   ,  \"τS\" -> 0.000000000000   ,  \"τN\" -> 0.000000000000   ,  \"τC\" -> 0.000000000000   ,  \"κ0\" -> 0.000000000000   ,  \"mm1\" -> 0.000000000000   ,  \"mm2\" -> 0.000000000000   ,  \"mm3\" -> 0.000000000000   ,  \"T\" -> 0.120000000000   ,  \"B\" -> 4.000000000000   ,  \"θ\" -> 45.000000000000   ,  \"Reoff\" -> 0.000000000000   ,  \"Imoff\" -> 0.000000000000   ,  \"στ1\" -> 0.000000000000   ,  \"στS\" -> 0.000000000000   ,  \"στN\" -> 0.000000000000    |>   , \n\"IDS0527_220605_RAW_cal__ref_\" ->   <|    \"ζ\" -> 0.163587274330   ,  \"τ1\" -> 0.177723598175   ,  \"τS\" -> 0.024747362505   ,  \"τN\" -> 0.010499593471   ,  \"τC\" -> 0.000964995814   ,  \"κ0\" -> 0.000000001207   ,  \"mm1\" -> 0.000131851499   ,  \"mm2\" -> 0.027402099160   ,  \"mm3\" -> 0.192167552763   ,  \"T\" -> 0.250000000000   ,  \"B\" -> 4.000000000000   ,  \"θ\" -> 45.000000000000   ,  \"Reoff\" -> -21493877.551020443400   ,  \"Imoff\" -> 0.000000000000   ,  \"στ1\" -> 0.096620218228   ,  \"στS\" -> 0.000434999932   ,  \"στN\" -> 0.007322093866    |>   , \n\"IDS0527_220605_RAW_cal__sam_\" ->   <|    \"ζ\" -> 0.000000000000   ,  \"τ1\" -> 0.000000000000   ,  \"τS\" -> 0.000000000000   ,  \"τN\" -> 0.000000000000   ,  \"τC\" -> 0.000000000000   ,  \"κ0\" -> 0.000000000000   ,  \"mm1\" -> 0.000000000000   ,  \"mm2\" -> 0.000000000000   ,  \"mm3\" -> 0.000000000000   ,  \"T\" -> 0.250000000000   ,  \"B\" -> 4.000000000000   ,  \"θ\" -> 45.000000000000   ,  \"Reoff\" -> 0.000000000000   ,  \"Imoff\" -> 0.000000000000   ,  \"στ1\" -> 0.000000000000   ,  \"στS\" -> 0.000000000000   ,  \"στN\" -> 0.000000000000    |>   , \n\"IDS0528_220605_RAW_cal__ref_\" ->   <|    \"ζ\" -> 0.115342924881   ,  \"τ1\" -> 0.183028972039   ,  \"τS\" -> 0.022615118092   ,  \"τN\" -> 0.006941794186   ,  \"τC\" -> 0.001037906865   ,  \"κ0\" -> 0.000000001545   ,  \"mm1\" -> 0.000103500075   ,  \"mm2\" -> 0.024936932480   ,  \"mm3\" -> 0.191992539340   ,  \"T\" -> 0.300000000000   ,  \"B\" -> 4.000000000000   ,  \"θ\" -> 45.000000000000   ,  \"Reoff\" -> -13363265.306122444600   ,  \"Imoff\" -> 0.000000000000   ,  \"στ1\" -> 0.063499413801   ,  \"στS\" -> 0.000291757985   ,  \"στN\" -> 0.002527808179    |>   , \n\"IDS0528_220605_RAW_cal__sam_\" ->   <|    \"ζ\" -> 0.000000000000   ,  \"τ1\" -> 0.000000000000   ,  \"τS\" -> 0.000000000000   ,  \"τN\" -> 0.000000000000   ,  \"τC\" -> 0.000000000000   ,  \"κ0\" -> 0.000000000000   ,  \"mm1\" -> 0.000000000000   ,  \"mm2\" -> 0.000000000000   ,  \"mm3\" -> 0.000000000000   ,  \"T\" -> 0.300000000000   ,  \"B\" -> 4.000000000000   ,  \"θ\" -> 45.000000000000   ,  \"Reoff\" -> 0.000000000000   ,  \"Imoff\" -> 0.000000000000   ,  \"στ1\" -> 0.000000000000   ,  \"στS\" -> 0.000000000000   ,  \"στN\" -> 0.000000000000    |>   , \n\"IDS0529_220605_RAW_cal__ref_\" ->   <|    \"ζ\" -> 0.082205302754   ,  \"τ1\" -> 0.199068291340   ,  \"τS\" -> 0.021395603563   ,  \"τN\" -> 0.004747138238   ,  \"τC\" -> 0.001295613399   ,  \"κ0\" -> 0.000000001948   ,  \"mm1\" -> 0.000093558415   ,  \"mm2\" -> 0.023663557896   ,  \"mm3\" -> 0.204898602234   ,  \"T\" -> 0.360000000000   ,  \"B\" -> 4.000000000000   ,  \"θ\" -> 45.000000000000   ,  \"Reoff\" -> -6702040.816326528790   ,  \"Imoff\" -> 0.000000000000   ,  \"στ1\" -> 0.038070369381   ,  \"στS\" -> 0.000151057018   ,  \"στN\" -> 0.001245904687    |>   , \n\"IDS0529_220605_RAW_cal__sam_\" ->   <|    \"ζ\" -> 0.000000000000   ,  \"τ1\" -> 0.000000000000   ,  \"τS\" -> 0.000000000000   ,  \"τN\" -> 0.000000000000   ,  \"τC\" -> 0.000000000000   ,  \"κ0\" -> 0.000000000000   ,  \"mm1\" -> 0.000000000000   ,  \"mm2\" -> 0.000000000000   ,  \"mm3\" -> 0.000000000000   ,  \"T\" -> 0.360000000000   ,  \"B\" -> 4.000000000000   ,  \"θ\" -> 45.000000000000   ,  \"Reoff\" -> 0.000000000000   ,  \"Imoff\" -> 0.000000000000   ,  \"στ1\" -> 0.000000000000   ,  \"στS\" -> 0.000000000000   ,  \"στN\" -> 0.000000000000    |>   , \n\"IDS0530_220605_RAW_cal__ref_\" ->   <|    \"ζ\" -> 0.062434773086   ,  \"τ1\" -> 0.091033034747   ,  \"τS\" -> 0.021000801063   ,  \"τN\" -> 0.002166413652   ,  \"τC\" -> 0.001607646673   ,  \"κ0\" -> 0.000000002334   ,  \"mm1\" -> 0.000088451406   ,  \"mm2\" -> 0.023050943702   ,  \"mm3\" -> 0.094114940821   ,  \"T\" -> 0.420000000000   ,  \"B\" -> 4.000000000000   ,  \"θ\" -> 45.000000000000   ,  \"Reoff\" -> -3579591.836734689770   ,  \"Imoff\" -> 0.000000000000   ,  \"στ1\" -> 0.001625101640   ,  \"στS\" -> 0.000103039832   ,  \"στN\" -> 0.000006624579    |>   , \n\"IDS0530_220605_RAW_cal__sam_\" ->   <|    \"ζ\" -> 0.000000000000   ,  \"τ1\" -> 0.000000000000   ,  \"τS\" -> 0.000000000000   ,  \"τN\" -> 0.000000000000   ,  \"τC\" -> 0.000000000000   ,  \"κ0\" -> 0.000000000000   ,  \"mm1\" -> 0.000000000000   ,  \"mm2\" -> 0.000000000000   ,  \"mm3\" -> 0.000000000000   ,  \"T\" -> 0.420000000000   ,  \"B\" -> 4.000000000000   ,  \"θ\" -> 45.000000000000   ,  \"Reoff\" -> 
